vi "HV Load V_Settings.vi"() -> (0 "appended path":path, 2 "Number of PMTs":i32, 3 "V_Settings":string[][](array[string]))   [LabVIEW 2018, in "HV QMH.lvlib"]
uses:
  HV QMH.lvlib
  <vilib>/Utility/file.llb/Read Delimited Spreadsheet (string).vi
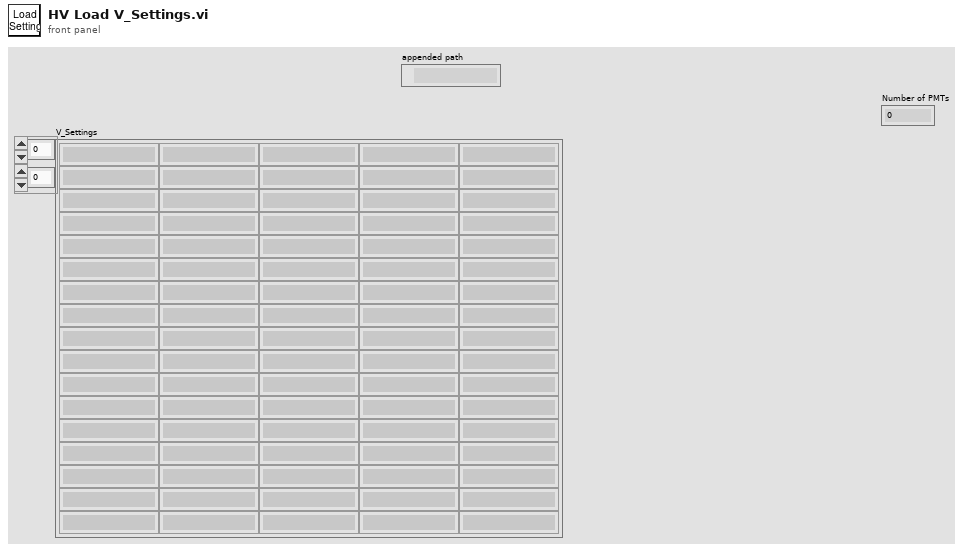
[diagram p1: front panel]
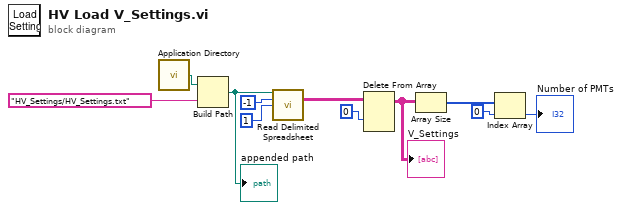
[diagram p0: block diagram]
diagram:
  n1 = call <vilib>:"Application Directory.vi"() -> ("Application Directory"=w5:path)
  n2 = Build Path(base path=w5, name or relative path="HV_Settings/HV_Settings.txt") -> (appended path=w7:path)
  "appended path" <- w7
  n3 = call-poly <vilib>:"Read Delimited Spreadsheet.vi"("file path (dialog if empty)"=w7, "number of rows (all:-1)"=-1, "start of read offset (chars.:0)"=1) -> ("all rows"=w10:string[][])  [unwired: 7 in, 5 out]
  n4 = Delete From Array(array=w10, index (row)=0) -> (array with subset deleted=w4:string[][])  [unwired: 2 in, 1 out]
  "V_Settings" <- w4
  n5 = Array Size(array=w4) -> (size(s)=w3:i32[])
  n6 = Index Array(array=w3, index=0) -> (element=→"Number of PMTs":i32)
